vi "Read ProcRepo.vi"(8 "error in (no error)":errorcluster, 11 "SetListPrefs in":refnum<class "SetListPrefs.lvclass">) -> (0 "error out":errorcluster, 2 "ProcRepo":path, 3 "SetListPrefs out":refnum<class "SetListPrefs.lvclass">)   [LabVIEW 2013, in "SetListPrefs.lvclass"]
uses:
  SetListPrefs.lvclass
  SetListPrefs.lvclass/SetListPrefs.ctl
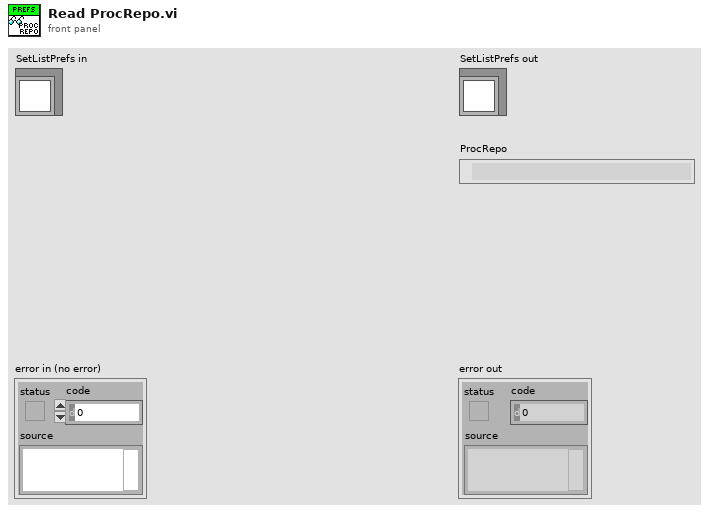
[diagram p1: front panel]
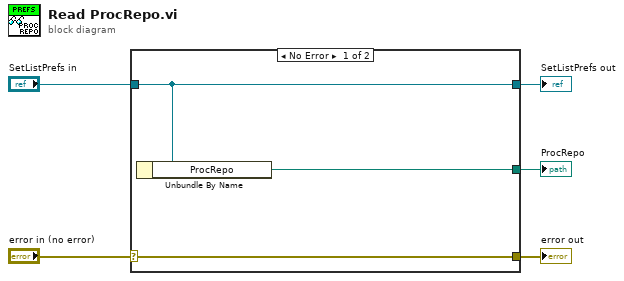
[diagram p0: block diagram]
diagram:
  n1 = case shown="No Error" "error in (no error)" {
    selector: "error in (no error)" -> [w8 w9]
    tunnel: [w8 w9] -> w4
    tunnel: [w7 w10] -> w2
    tunnel: "SetListPrefs in" -> [w7 w10]
    tunnel: [w6 _] -> w1
    frame No Error {
      n2 = Unbundle By Name(w7) -> ("ProcRepo"=w6:path)
    }
    frame Error {
    }
  }
  "error out" <- w4
  "SetListPrefs out" <- w2
  "ProcRepo" <- w1
